vi "Build Motion.vi"(6 "Type":enum16{"Relative", "Absolute"}(ring)=enum."Absolute", 7 "Speed Limit":refnum<class "Vec3d Class.lvclass">, 8 "error in":errorcluster, 9 "Speed":dbl, 10 "End/Offset":refnum<class "Vec3d Class.lvclass">, 11 "Start":refnum<class "Vec3d Class.lvclass">) -> (0 "error out":errorcluster, 1 "Axes":string[](array[string]), 2 "Speeds":dbl[](array[numeric]), 3 "End/Offset":dbl[](array[numeric]))   [LabVIEW 2011]
uses:
  Vec3d Class/Vec3d Class.lvclass
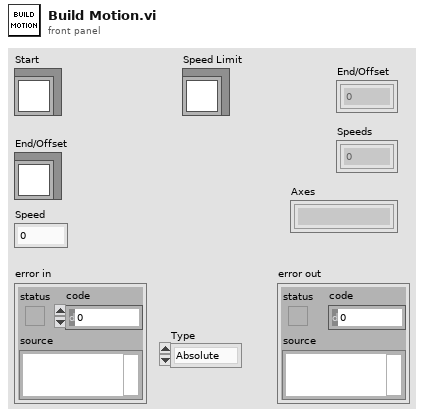
[diagram p1: front panel]
types:
  T1 = cluster{"Axis":string, "Coordinate":dbl, "Speed":dbl}[]
  T2 = cluster{"Axis":string, "Coordinate":dbl, "Speed":dbl}
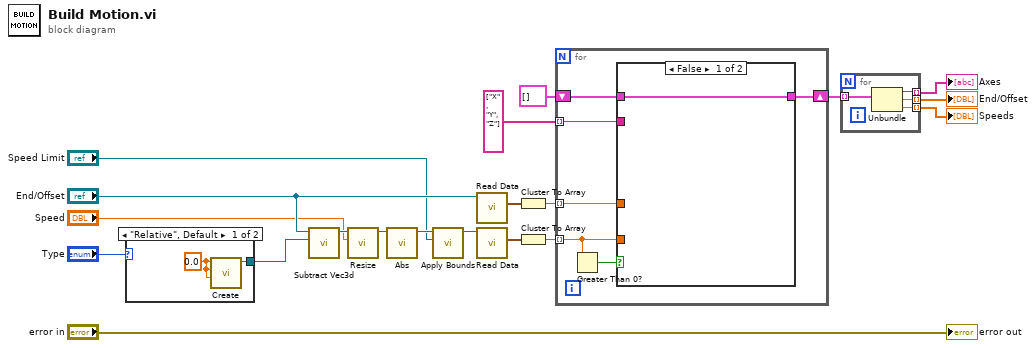
[diagram p0: block diagram]
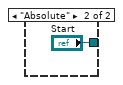
[diagram p2: hidden frame]
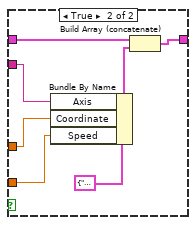
[diagram p3: hidden frame]
diagram:
  n1 = case shown="\"Relative\", Default" "Type" {
    tunnel: [w21 "Start"] -> w9
    frame "Relative", Default {
      w22 = 0.0 ("X")
      n2 = call "Create.vi"("Z"=w22, "Y"=w22, "X"=w22) -> ("Vec3d Class out"=w21:refnum<class "Vec3d Class.lvclass">)  [unwired: 7 in, 1 out]
    }
    frame "Absolute" {
    }
  }
  n3 = call "Subtract Vec3d.vi"("Vec3d in 2"=w9, "Vec3d in 1"="End/Offset") -> ("Vec3d Class out"=w12:refnum<class "Vec3d Class.lvclass">)  [unwired: 8 in, 1 out]
  n4 = call "Resize.vi"("length"="Speed", "Vec3d in"=w12) -> ("Vec3d out"=w11:refnum<class "Vec3d Class.lvclass">)  [unwired: 8 in, 1 out]
  n5 = call "Abs.vi"("Vec3d in"=w11) -> ("Vec3d out"=w3:refnum<class "Vec3d Class.lvclass">)  [unwired: 9 in, 1 out]
  n6 = call "Apply Bounds.vi"("Bounds"="Speed Limit", "Vec3d in"=w3) -> ("Vec3d out"=w1:refnum<class "Vec3d Class.lvclass">)  [unwired: 8 in, 1 out]
  n7 = call-dynamic "Read Data.vi"("Vec3d Class in"="End/Offset") -> ("Data"=w20:cluster{"X":dbl, "Y":dbl, "Z":dbl})  [unwired: 8 in, 2 out]
  n8 = call-dynamic "Read Data.vi"("Vec3d Class in"=w1) -> ("Data"=w7:cluster{"X":dbl, "Y":dbl, "Z":dbl})  [unwired: 8 in, 2 out]
  n9 = Cluster To Array(cluster=w20) -> (array=w18:dbl[])
  n10 = Cluster To Array(cluster=w7) -> (array=w6:dbl[])
  n11 = for {
    tunnel: string[] ["X", "Y", "Z"] -> [w29] mode=indexing
    tunnel: w18 -> [w28] mode=indexing
    shift-right: [w27] -> w15
    shift-left: T1 [] -> [w26]
    tunnel: w6 -> [w24] mode=indexing
    n12 = Greater Than 0?(x=w24) -> (x > 0?=w25:bool)
    n13 = case shown="False" w25 {
      tunnel: w29 -> [_ w36]
      tunnel: w28 -> [_ w37]
      tunnel: [w30 w33] -> w27
      tunnel: w26 -> [w30 w35]
      tunnel: w24 -> [_ w31]
      frame False {
      }
      frame True {
        n14 = Bundle By Name(cluster=T2 {"Axis"="", "Coordinate"=0.0, "Speed"=0.0}, "Axis"=w36, "Coordinate"=w37, "Speed"=w31) -> (w34:T2)
        n15 = Build Array (concatenate)(w35, w34) -> (w33:T1)
      }
    }
  }
  n16 = for {
    tunnel: w15 -> [w41] mode=indexing
    tunnel: [w40] -> w14 mode=indexing
    tunnel: [w39] -> w13 mode=indexing
    tunnel: [w38] -> w4 mode=indexing
    n17 = Unbundle(w41) -> ("Axis"=w40:string, "Coordinate"=w39:dbl, "Speed"=w38:dbl)
  }
  "Axes" <- w14
  "End/Offset" <- w13
  "Speeds" <- w4
  "error out" <- "error in"
